vi "Config Hardware.vi"(8 "error in (no error)":errorcluster, 11 "System Modules Factory in":refnum<class "System Modules Factory.lvclass">) -> (0 "error out":errorcluster, 3 "System Modules Factory out":refnum<class "System Modules Factory.lvclass">)   [LabVIEW 2019, in "System Modules Factory.lvclass"]
uses:
  System Modules Factory.lvclass
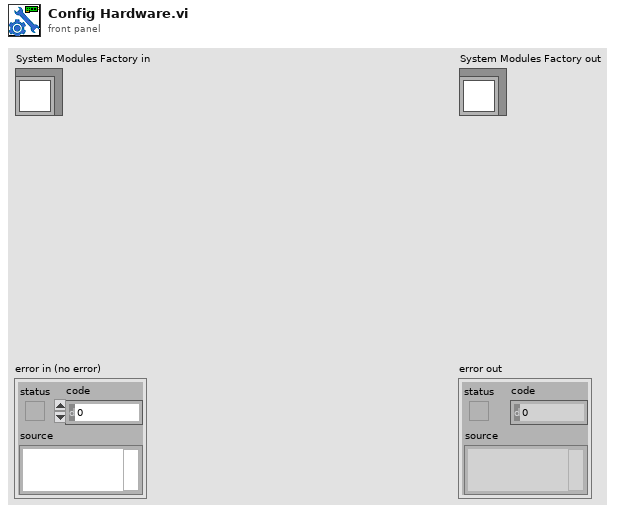
[diagram p1: front panel]
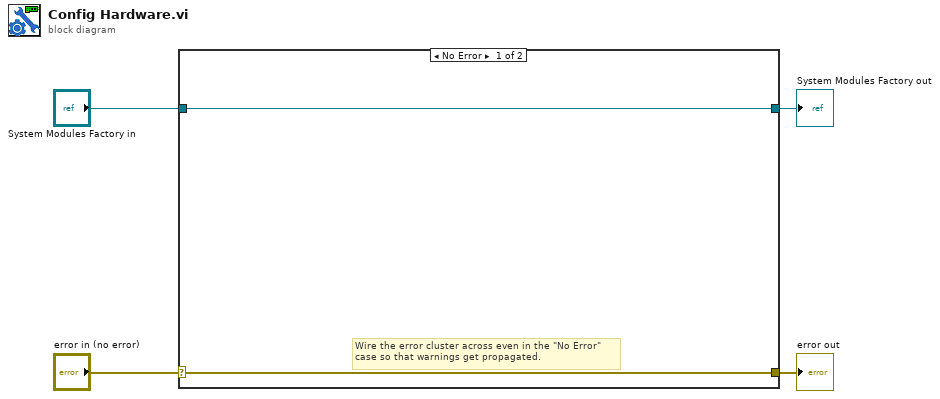
[diagram p0: block diagram]
diagram:
  n1 = case shown="No Error" "error in (no error)" {
    selector: "error in (no error)" -> [w5 w8]
    tunnel: [w5 w8] -> w3
    tunnel: [w6 w7] -> w1
    tunnel: "System Modules Factory in" -> [w6 w7]
    frame No Error {
      # "Wire the error cluster across even in the \"No Error\"\ncase so that warnings get propagated."
    }
    frame Error {
    }
  }
  "error out" <- w3
  "System Modules Factory out" <- w1
